vi "SNMP Variable.vi"() -> ()   [LabVIEW 2010]
panel:
  out "SNMP Array":dbl[](array[numeric])
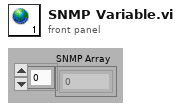
[diagram p1: front panel]
diagram:
